vi "Procesado_Bidirec_fotoc_aRMS.vi"(0 "Paths_canales_aRMS":path[](array[path]), 1 "Distancias generales (m)":dbl[](array[numeric]), 2 "Distancias\nacelerometros":dbl[](array[numeric]), 3 "Ejes Procesados":i32, 5 "Paths_canales_aRMS 2":path[](array[path]), 6 "dt RMS 2":dbl, 7 "Distancias centrales de las ruedas\n               configuración (m)":dbl[](array[numeric]), 8 "Puntos 2":sgl[](array[numeric]), 9 "Parámetros acelerómetros":dbl[](array[numeric]), 10 "Frecuencia de muestreo":dbl, 11 "Puntos":sgl[](array[numeric])) -> (4 "Max RMS Ruedas":dbl[][](array[numeric]))   [LabVIEW 2015]
uses:
  <vilib>/Analysis/3filter.llb/Filter Passband Type.ctl
  <vilib>/Analysis/5stat.llb/RMS (DBL).vi
  <vilib>/Analysis/3filter.llb/Butterworth Filter (DBL).vi
  <vilib>/measure/madcrms.llb/Basic Averaged DC-RMS for 1 Chan.vi
  <vilib>/measure/NI_MAPro.lvlib
  <vilib>/Analysis/NI_AALBase.lvlib
  <vilib>/Analysis/NI_AALPro.lvlib
panel:
  out "Max RMS Ruedas 2":dbl[][](array[numeric])
  out "Waveform Graph 2":dbl[](graph)
  out "Waveform Graph":dbl[](graph)
  out "dt RMS":dbl
  out "Loop Rate (Hz)":dbl
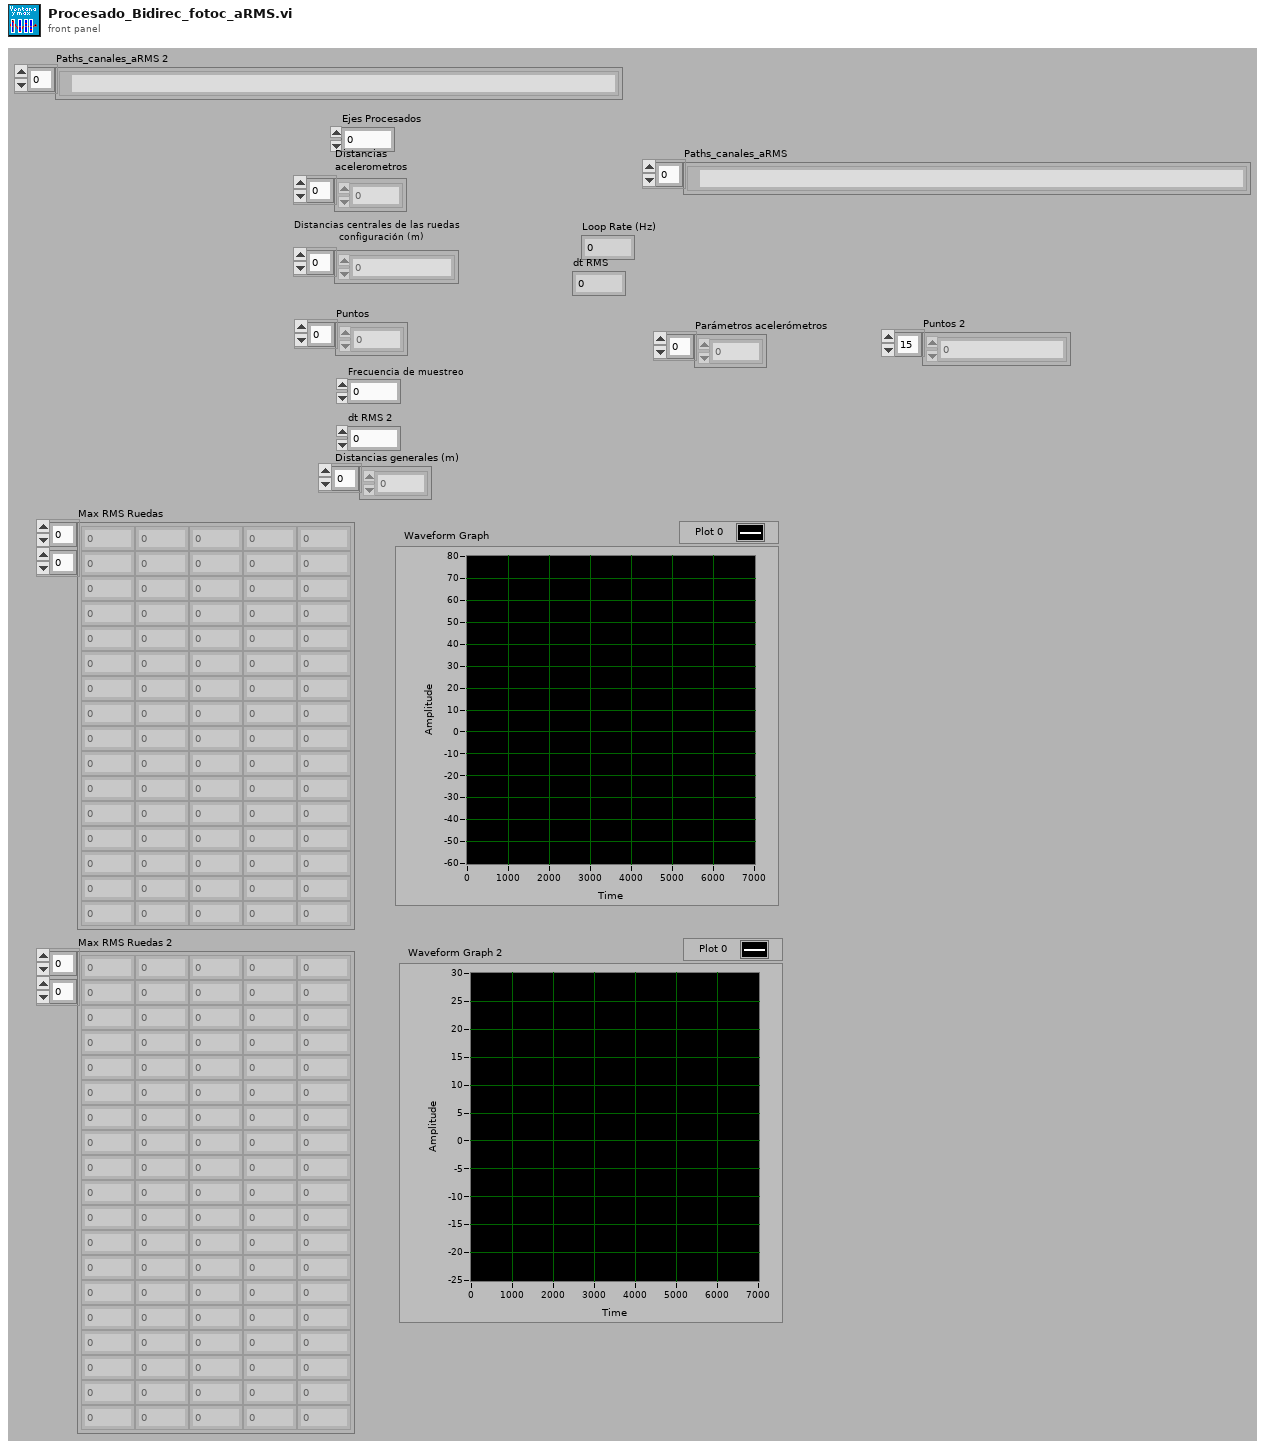
[diagram p1: front panel]
types:
  T1 = typedef "NI_AALBase.lvlib/Filter Passband Type.ctl" = enum32{"Lowpass", "Highpass", "Bandpass", "Bandstop"}
  T2 = enum16{"big-endian, network order", "native, host order", "little-endian"}
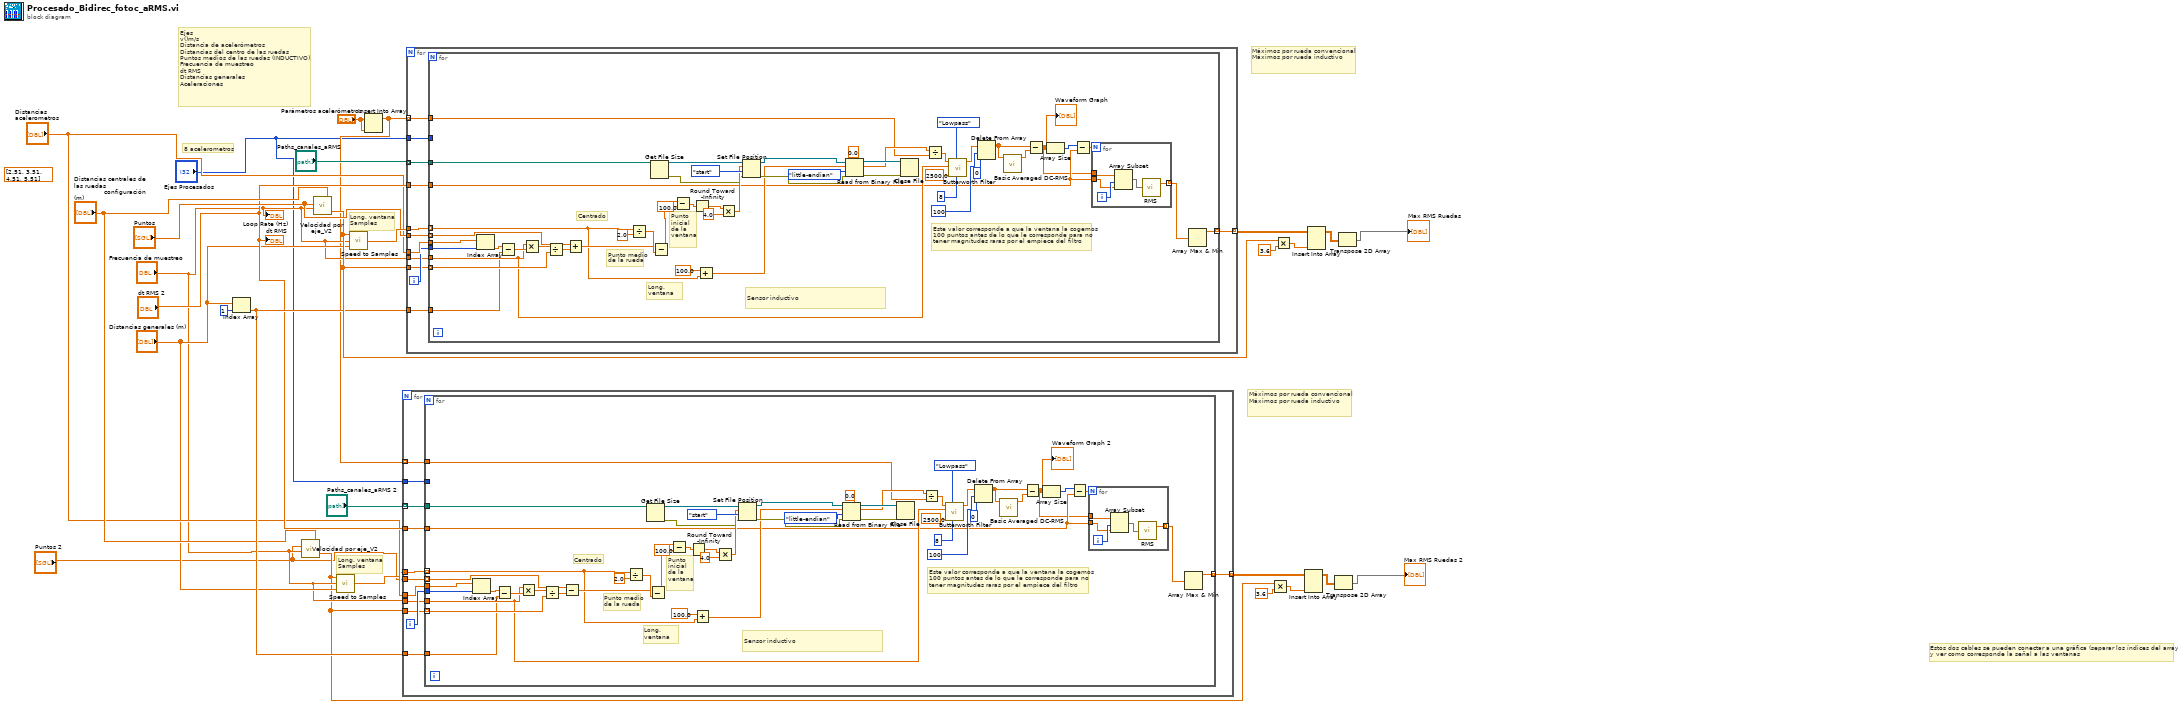
[diagram p0: block diagram]
diagram:
  (unwired) dbl[] [2.51, 3.51, 4.51, 5.51] ("Distancias\nacelerometros")
  # "Long. ventana\nSamples"
  # "Máximos por rueda convencional\nMáximos por rueda inductivo"
  # "Long. ventana\nSamples"
  # "8 acelerometros"
  # "Ejes\nv()m/s\nDistancia de acelerómetros\nDistancias del centro de las ruedas\nPuntos medios de las ruedas (INDUCTIVO)\nFrecuencia de muestreo\ndt RMS\nDistancias generales\nAceleraciones"
  # "Máximos por rueda convencional\nMáximos por rueda inductivo"
  # "Estos dos cables se pueden conectar a una gráfica (separar los índices del array)\ny ver como corresponde la señal a las ventanas"
  n1 = Index Array(array="Distancias generales (m)", index=1) -> (element=w11:dbl)
  n2 = call "Velocidad por eje_V2.vi"("Distancias centrales de las ruedas\n               configuración (m)"="Distancias centrales de las ruedas\n               configuración (m)", "Frecuencia de muestreo"="Frecuencia de muestreo", "Puntos centrales de las ruedas\n             inductivo"="Puntos 2") -> ("Velocidad de eje"=w2:dbl[])  [unwired: 2 in]
  n3 = call "Velocidad por eje_V2.vi"("Distancias centrales de las ruedas\n               configuración (m)"="Distancias centrales de las ruedas\n               configuración (m)", "Frecuencia de muestreo"="Frecuencia de muestreo", "Puntos centrales de las ruedas\n             inductivo"="Puntos") -> ("Velocidad de eje"=w25:dbl[])  [unwired: 2 in]
  n4 = call "Speed to Samples.vi"("Distancias generales (m)"="Distancias generales (m)", "Loop Rate (Hz)"="Frecuencia de muestreo", "Velocidad de eje(m/s)"=w2) -> ("Longitud de ventana (puntos)"=w5:dbl[])
  n5 = call "Speed to Samples.vi"("Distancias generales (m)"="Distancias generales (m)", "Loop Rate (Hz)"="Frecuencia de muestreo", "Velocidad de eje(m/s)"=w25) -> ("Longitud de ventana (puntos)"=w28:dbl[])
  n6 = Insert Into Array(array="Parámetros acelerómetros", new element="Parámetros acelerómetros") -> (w4:dbl[])  [unwired: 1 in]
  n7 = for {
    tunnel: w5 -> [w30]
    tunnel: "Puntos 2" -> [w38]
    tunnel: w2 -> [w35]
    tunnel: "Distancias\nacelerometros" -> [w39]
    tunnel: "dt RMS 2" -> [w40]
    tunnel: [w37] -> w17 mode=indexing
    tunnel: "Ejes Procesados" -> [w31]
    tunnel: "Frecuencia de muestreo" -> [w32]
    tunnel: "Paths_canales_aRMS 2" -> [w34] mode=indexing
    tunnel: w4 -> [w33] mode=indexing
    tunnel: w11 -> [w29]
    i -> [w36]
    n8 = for {
      tunnel: w40 -> [w44]
      tunnel: w39 -> [w88]
      tunnel: w38 -> [w87] mode=indexing
      tunnel: [w86] -> w37 mode=indexing
      tunnel: w36 -> [w85]
      tunnel: w35 -> [w84] mode=indexing
      tunnel: w34 -> [w68]
      tunnel: w33 -> [w78]
      tunnel: w32 -> [w59]
      tunnel: w31 -> [_]
      tunnel: w30 -> [w55] mode=indexing
      tunnel: w29 -> [w43]
      # "Este valor corresponde a que la ventana la cogemos\n100 puntos antes de lo que le corresponde para no \ntener magnitudes raras por el empiece del filtro"
      # "Centrado"
      # "Sensor inductivo"
      # "Long.\nventana"
      # "Punto\ninicial\nde la \nventana"
      # "Punto medio\nde la rueda"
      n9 = Index Array(array=w88, index=w85) -> (element=w74:dbl)
      n10 = Subtract(x=w74, y=w43) -> (x-y=w71:dbl)
      n11 = Multiply(x=w59, y=w71) -> (x*y=w73:dbl)
      n12 = Divide(x=w73, y=w84) -> (x/y=w72:dbl)
      n13 = Subtract(x=w87, y=w72) -> (x-y=w60:dbl)
      n14 = Divide(x=w55, y=2.0) -> (x/y=w69:dbl)
      n15 = Get File Size(file=w68) -> (refnum out=w66:refnum<file>, 0:w62:errorcluster)  [unwired: 1 in, 1 out]
      n16 = Subtract(x=w60, y=w69) -> (x-y=w48:dbl)
      n17 = Subtract(x=w48, y=100.0 ("x")) -> (x-y=w57:dbl)
      n18 = Round Toward -Infinity(1:w57) -> (0:w58:dbl)
      n19 = Add(x=100.0, y=w55) -> (x+y=w54:dbl)
      n20 = Multiply(x=w58, y=4.0) -> (x*y=w64:dbl)
      n21 = Set File Position(offset (in bytes) (0)=w64, refnum=w66, from (0:start)=enum16{"start", "end", "current"}."start", error in=w62) -> (refnum out=w63:refnum<file>, error out=w61:errorcluster)
      n22 = Read from Binary File(5:sgl 0.0, 8:w61, 9:T2."little-endian" ("byte order (0:big-endian, network order)"), 10:w54, 11:w63) -> (0:w82:errorcluster, 2:w79:sgl[], 3:w83:refnum<file>)  [unwired: 2 out]
      n23 = Close File(refnum=w83, error in=w82) -> ()  [unwired: 2 out]
      n24 = Divide(x=w79, y=w78) -> (x/y=w75:dbl[])
      n25 = call-poly <vilib>:"Butterworth Filter.vi"("order"=8, "filter type"=Filter_Passband_Type."Lowpass", "low cutoff freq: fl"=2500.0, "sampling freq: fs"=w59, "X"=w75) -> ("Filtered X"=w53:dbl[])  [unwired: 3 in, 1 out]
      n26 = Delete From Array(array=w53, length=100, index=0) -> (array with subset deleted=w52:dbl[])  [unwired: 1 out]
      n27 = call-poly <vilib>:"Basic Averaged DC-RMS.vi"("signal in"=w52) -> ("DC value"=w89:dbl)  [unwired: 4 in, 6 out]
      n28 = Subtract(x=w52, y=w89) -> (x-y=w41:dbl[])
      "Waveform Graph 2" <- w41
      n29 = Array Size(array=w41) -> (size(s)=w45:i32)
      n30 = Subtract(x=w45, y=w44) -> (x-y=w46:dbl)
      n31 = for {
        N: w46 -> [_]
        tunnel: w44 -> [w91]
        tunnel: [w94] -> w42 mode=indexing
        tunnel: w41 -> [w93]
        i -> [w92]
        n32 = Array Subset(array=w93, index=w92, length=w91) -> (w90:dbl[])
        n33 = call-poly <vilib>:"RMS.vi"("X"=w90) -> ("rms value"=w94:dbl)  [unwired: 1 out]
      }
      n34 = Array Max & Min(array=w42) -> (max value=w86:dbl)  [unwired: 3 out]
    }
  }
  n35 = for {
    tunnel: w28 -> [w96]
    tunnel: "Puntos" -> [w104]
    tunnel: w25 -> [w101]
    tunnel: "Distancias\nacelerometros" -> [w105]
    tunnel: "dt RMS 2" -> [w106]
    tunnel: [w103] -> w26 mode=indexing
    tunnel: "Ejes Procesados" -> [w97]
    tunnel: "Frecuencia de muestreo" -> [w98]
    tunnel: "Paths_canales_aRMS" -> [w100] mode=indexing
    tunnel: w4 -> [w99] mode=indexing
    tunnel: w11 -> [w95]
    i -> [w102]
    n36 = for {
      tunnel: w106 -> [w110]
      tunnel: w105 -> [w154]
      tunnel: w104 -> [w153] mode=indexing
      tunnel: [w152] -> w103 mode=indexing
      tunnel: w102 -> [w151]
      tunnel: w101 -> [w150] mode=indexing
      tunnel: w100 -> [w134]
      tunnel: w99 -> [w144]
      tunnel: w98 -> [w125]
      tunnel: w97 -> [_]
      tunnel: w96 -> [w121] mode=indexing
      tunnel: w95 -> [w109]
      # "Este valor corresponde a que la ventana la cogemos\n100 puntos antes de lo que le corresponde para no \ntener magnitudes raras por el empiece del filtro"
      # "Centrado"
      # "Sensor inductivo"
      # "Long.\nventana"
      # "Punto\ninicial\nde la \nventana"
      # "Punto medio\nde la rueda"
      n37 = Index Array(array=w154, index=w151) -> (element=w140:dbl)
      n38 = Subtract(x=w140, y=w109) -> (x-y=w137:dbl)
      n39 = Multiply(x=w125, y=w137) -> (x*y=w139:dbl)
      n40 = Divide(x=w139, y=w150) -> (x/y=w138:dbl)
      n41 = Add(x=w153, y=w138) -> (x+y=w126:dbl)
      n42 = Divide(x=w121, y=2.0) -> (x/y=w135:dbl)
      n43 = Get File Size(file=w134) -> (refnum out=w132:refnum<file>, 0:w128:errorcluster)  [unwired: 1 in, 1 out]
      n44 = Subtract(x=w126, y=w135) -> (x-y=w114:dbl)
      n45 = Subtract(x=w114, y=100.0 ("x")) -> (x-y=w123:dbl)
      n46 = Round Toward -Infinity(1:w123) -> (0:w124:dbl)
      n47 = Add(x=100.0, y=w121) -> (x+y=w120:dbl)
      n48 = Multiply(x=w124, y=4.0) -> (x*y=w130:dbl)
      n49 = Set File Position(offset (in bytes) (0)=w130, refnum=w132, from (0:start)=enum16{"start", "end", "current"}."start", error in=w128) -> (refnum out=w129:refnum<file>, error out=w127:errorcluster)
      n50 = Read from Binary File(5:sgl 0.0, 8:w127, 9:T2."little-endian" ("byte order (0:big-endian, network order)"), 10:w120, 11:w129) -> (0:w148:errorcluster, 2:w145:sgl[], 3:w149:refnum<file>)  [unwired: 2 out]
      n51 = Close File(refnum=w149, error in=w148) -> ()  [unwired: 2 out]
      n52 = Divide(x=w145, y=w144) -> (x/y=w141:dbl[])
      n53 = call-poly <vilib>:"Butterworth Filter.vi"("order"=8, "filter type"=Filter_Passband_Type."Lowpass", "low cutoff freq: fl"=2500.0, "sampling freq: fs"=w125, "X"=w141) -> ("Filtered X"=w119:dbl[])  [unwired: 3 in, 1 out]
      n54 = Delete From Array(array=w119, length=100, index=0) -> (array with subset deleted=w118:dbl[])  [unwired: 1 out]
      n55 = call-poly <vilib>:"Basic Averaged DC-RMS.vi"("signal in"=w118) -> ("DC value"=w155:dbl)  [unwired: 4 in, 6 out]
      n56 = Subtract(x=w118, y=w155) -> (x-y=w107:dbl[])
      "Waveform Graph" <- w107
      n57 = Array Size(array=w107) -> (size(s)=w111:i32)
      n58 = Subtract(x=w111, y=w110) -> (x-y=w112:dbl)
      n59 = for {
        N: w112 -> [_]
        tunnel: w110 -> [w157]
        tunnel: [w160] -> w108 mode=indexing
        tunnel: w107 -> [w159]
        i -> [w158]
        n60 = Array Subset(array=w159, index=w158, length=w157) -> (w156:dbl[])
        n61 = call-poly <vilib>:"RMS.vi"("X"=w156) -> ("rms value"=w160:dbl)  [unwired: 1 out]
      }
      n62 = Array Max & Min(array=w108) -> (max value=w152:dbl)  [unwired: 3 out]
    }
  }
  n63 = Multiply(x=w2, y=3.6) -> (x*y=w15:dbl[])
  n64 = Multiply(x=w25, y=3.6) -> (x*y=w23:dbl[])
  n65 = Insert Into Array(array=w17, new element=w15) -> (w14:dbl[][])  [unwired: 2 in]
  n66 = Insert Into Array(array=w26, new element=w23) -> (w19:dbl[][])  [unwired: 2 in]
  n67 = Transpose 2D Array(2D array=w14) -> (transposed array=→"Max RMS Ruedas 2":dbl[][])
  n68 = Transpose 2D Array(2D array=w19) -> (transposed array=→"Max RMS Ruedas":dbl[][])
  "Loop Rate (Hz)" <- "Frecuencia de muestreo"
  "dt RMS" <- "dt RMS 2"
